vi "Measure.vi"(8 "error in (no error)":errorcluster, 9 "measurement configuration":variant, 10 "measure call context in":refnum<class "Measure Call Context.lvclass">, 11 "measurement plugin in":refnum<class "FPT_SParam_VST.lvclass">) -> (0 "error out":errorcluster, 1 "measurement results":variant, 2 "measure call context out":refnum<class "Measure Call Context.lvclass">, 3 "measurement plugin out":refnum<class "FPT_SParam_VST.lvclass">)   [LabVIEW 2023, in "FPT_SParam_VST.lvclass"]
uses:
  FPT_SParam_VST.lvclass
  <vilib>/Plug-In SDKs/Measurements/Measure Call Context/Measure Call Context.lvclass
  Measurement Configuration.ctl
  FPT_SParam_VST.lvclass/FPT_SParam_VST.ctl
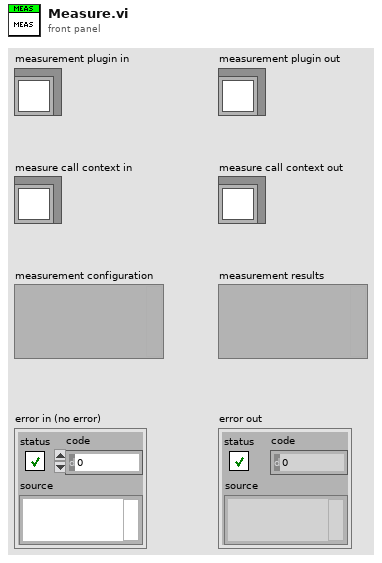
[diagram p1: front panel]
types:
  T1 = typedef "FPT_SParam_VST.lvclass/Measurement Configuration.ctl" = cluster{"Automation Test":bool, "Power sequencing file path":string, "VST Resource Name":string, "RFSG port":string, "RFmx port":string, "RF Out Switch":string, "Common RFout":string, "Port1 Incident":string, "Port2 Incident":string, "RF In Switch":string, "Common RFin":string, "Port1 Reference":string, "Port1 Test":string, "Port2 Reference":string, "Port2 Test":string, "RFSG attenuation mode":enum32{"<None>", "Constant Attenuation"}, "RFSG external attenuation (dB)":dbl, "Save Calibration File at":string, "Short S1P":string, "Open S1P":string, "Load S1P":string, "Through Adapter S2P":string, "Action":enum32{"Calibrate", "Measure"}, "Power Level (dBm)":dbl, "External Gain (dB)":dbl, "Start Frequency (Hz)":dbl, "Stop Frequency (Hz)":dbl, "Step Size (Hz)":dbl, "Type of Stimulus":enum32{"CW", "Pulsed CW"}, "Pulse Width (s)":dbl, "PRI (s)":dbl, "IF Bandwidth (Hz)":dbl, "Average Mode":enum32{"Per Sweep", "Per Point"}, "Number of Averages":i32, "SnP File Path":string, "Calibration File Path":string, "Power sequencing file validity check":bool}
  T2 = typedef "FPT_SParam_VST.lvclass/Measurement Results.ctl" = cluster{"Status":string, "S-Param Magnitude":dbl[][], "S-Param Phase":dbl[][], "S21 (Mean)":dbl, "S12 (Mean)":dbl}
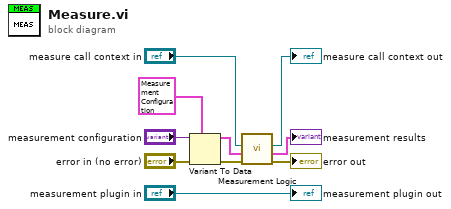
[diagram p0: block diagram]
diagram:
  n1 = Variant To Data(error in="error in (no error)", type=T1 {"Automation Test"=FALSE, "Power sequencing file path"="Lorem ipsum dolor sit", "VST Resource Name"="5842_0", "RFSG port"="", "RFmx port"="", "RF Out Switch"="", "Common RFout"="", "Port1 Incident"="", "Port2 Incident"="", "RF In Switch"="", "Common RFin"="", "Port1 Reference"="", "Port1 Test"="", "Port2 Reference"="", "Port2 Test"="", "RFSG attenuation mode"=enum."Constant Attenuation", "RFSG external attenuation (dB)"=1.0, "Save Calibration File at"="", "Short S1P"="", "Open S1P"="", "Load S1P"="", "Through Adapter S2P"="", "Action"=enum."Measure", "Power Level (dBm)"=1.0, "External Gain (dB)"=2e-05, "Start Frequency (Hz)"=4000000000.0, "Stop Frequency (Hz)"=26000000000.0, "Step Size (Hz)"=0.0, "Type of Stimulus"=enum."Pulsed CW", "Pulse Width (s)"=0.0, "PRI (s)"=0.0, "IF Bandwidth (Hz)"=1.0, "Average Mode"=enum."Per Sweep", "Number of Averages"=0, "SnP File Path"="", "Calibration File Path"="", "Power sequencing file validity check"=TRUE} ("measurement configuration"), Variant="measurement configuration") -> (data=w1:T1, error out=w7:errorcluster)
  n2 = call "Measurement Logic.vi"("error in"=w7, "measurement configuration"=w1, "measure call context in"="measure call context in") -> ("error out"=→"error out":errorcluster, "measurement results"=→"measurement results":T2, "measure call context out"=→"measure call context out":refnum<class "Measure Call Context.lvclass">)  [unwired: 6 in]
  "measurement plugin out" <- "measurement plugin in"
